vi "mul_add_24_dc_ht_rnd.vi"(8 "add":fxp<+/-,24,16> format="%#_10g", 10 "Signal":fxp<+/-,24,16>=32.0, 11 "coeff":fxp<+/-,18,2>=0.5) -> (1 "out":fxp<+/-,24,16>)   [LabVIEW 2018]
uses:
  <vilib>/rvi/FXPMathLib/basic elements/DSP48E/simVIs/niFpgaDsp48eSimulationState.ctl
  <vilib>/rvi/FXPMathLib/basic elements/DSP48E/subVIs/niFpgaDsp48eType.ctl
  <vilib>/rvi/FXPMathLib/basic elements/DSP48E/subVIs/niFpgaDsp48eAlumodeOpmodeCarryinselState.ctl
  <vilib>/rvi/FXPMathLib/basic elements/DSP48E/subVIs/niFpgaDsp48eUseMultiplierState.ctl
  <vilib>/rvi/FXPMathLib/basic elements/DSP48E/subVIs/niFpgaDsp48eLogicUnitModeState.ctl
  <vilib>/rvi/FXPMathLib/basic elements/DSP48E/subVIs/niFpgaDsp48eSelectPatternState.ctl
  <vilib>/rvi/FXPMathLib/basic elements/DSP48E/subVIs/niFpgaDsp48eSelectMaskState.ctl
  <vilib>/rvi/FXPMathLib/basic elements/DSP48E/subVIs/niFpgaDsp48eAutoresetState.ctl
  <vilib>/rvi/FXPMathLib/basic elements/DSP48E/simVIs/niFpgaDsp48eResets.ctl
  <vilib>/rvi/FXPMathLib/basic elements/DSP48E/simVIs/niFpgaDsp48eRegisters.ctl
  <vilib>/rvi/FXPMathLib/basic elements/DSP48E/simVIs/niFpgaDsp48eCheckMode.vi
  <vilib>/rvi/FXPMathLib/basic elements/DSP48E/simVIs/niFpgaDsp48eReportInvalidMode.vi
  <vilib>/rvi/FXPMathLib/basic elements/DSP48E/simVIs/niFpgaDsp48eSimBundleEnables.vi
  <vilib>/rvi/FXPMathLib/basic elements/DSP48E/simVIs/niFpgaDsp48eSimMultiplier.vi
  <vilib>/rvi/FXPMathLib/basic elements/DSP48E/simVIs/niFpgaDsp48eSimArithmetic.vi
  <vilib>/rvi/FXPMathLib/basic elements/DSP48E/simVIs/niFpgaDsp48eSimPatternDetect.vi
  <vilib>/rvi/FXPMathLib/basic elements/DSP48E/simVIs/niFpgaDsp48eSimP.vi
  <vilib>/rvi/FXPMathLib/basic elements/DSP48E/simVIs/niFpgaDsp48eSimUpdateState.vi
  <vilib>/rvi/FXPMathLib/basic elements/DSP48E/XNode/niFpgaDsp48e.xnode
panel:
  out "appended array 2":bool[](array[boolean])
  out "appended array":bool[](array[boolean])
  out "number":fxp<+/-,30,16>
  in  "Signal 2":fxp<+/-,24,16>=32.0
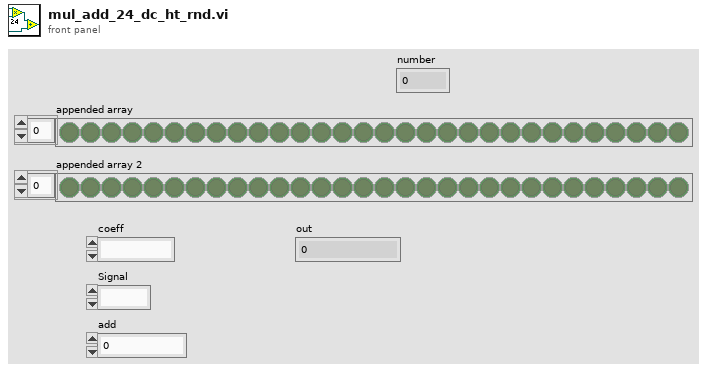
[diagram p1: front panel]
types:
  T1 = cluster{"Boolean array[0]":bool, "Boolean array[1]":bool, "Boolean array[2]":bool, "Boolean array[3]":bool, "Boolean array[4]":bool, "Boolean array[5]":bool, "Boolean array[6]":bool, "Boolean array[7]":bool, "Boolean array[8]":bool, "Boolean array[9]":bool, "Boolean array[10]":bool, "Boolean array[11]":bool, "Boolean array[12]":bool, "Boolean array[13]":bool, "Boolean array[14]":bool, "Boolean array[15]":bool, "Boolean array[16]":bool, "Boolean array[17]":bool, "Boolean array[18]":bool, "Boolean array[19]":bool, "Boolean array[20]":bool, "Boolean array[21]":bool, "Boolean array[22]":bool, "Boolean array[23]":bool}
  T2 = cluster{"Boolean array[0]":bool, "Boolean array[1]":bool, "Boolean array[2]":bool, "Boolean array[3]":bool, "Boolean array[4]":bool, "Boolean array[5]":bool, "Boolean array[6]":bool, "Boolean array[7]":bool, "Boolean array[8]":bool, "Boolean array[9]":bool, "Boolean array[10]":bool, "Boolean array[11]":bool, "Boolean array[12]":bool, "Boolean array[13]":bool, "Boolean array[14]":bool, "Boolean array[15]":bool, "Boolean array[16]":bool, "Boolean array[17]":bool}
  T3 = cluster{"Boolean array[0]":bool, "Boolean array[1]":bool, "Boolean array[2]":bool, "Boolean array[3]":bool, "Boolean array[4]":bool, "Boolean array[5]":bool, "Boolean array[6]":bool, "Boolean array[7]":bool, "Boolean array[8]":bool, "Boolean array[9]":bool, "Boolean array[10]":bool, "Boolean array[11]":bool, "Boolean array[12]":bool, "Boolean array[13]":bool, "Boolean array[14]":bool, "Boolean array[15]":bool, "Boolean array[16]":bool, "Boolean array[17]":bool, "Boolean array[18]":bool, "Boolean array[19]":bool, "Boolean array[20]":bool, "Boolean array[21]":bool, "Boolean array[22]":bool, "Boolean array[23]":bool, "Boolean array[24]":bool, "Boolean array[25]":bool, "Boolean array[26]":bool, "Boolean array[27]":bool, "Boolean array[28]":bool, "Boolean array[29]":bool, "Boolean array[30]":bool, "Boolean array[31]":bool, "Boolean array[32]":bool, "Boolean array[33]":bool, "Boolean array[34]":bool, "Boolean array[35]":bool, "Boolean array[36]":bool, "Boolean array[37]":bool, "Boolean array[38]":bool, "Boolean array[39]":bool, "Boolean array[40]":bool, "Boolean array[41]":bool, "Boolean array[42]":bool, "Boolean array[43]":bool, "Boolean array[44]":bool, "Boolean array[45]":bool, "Boolean array[46]":bool, "Boolean array[47]":bool}
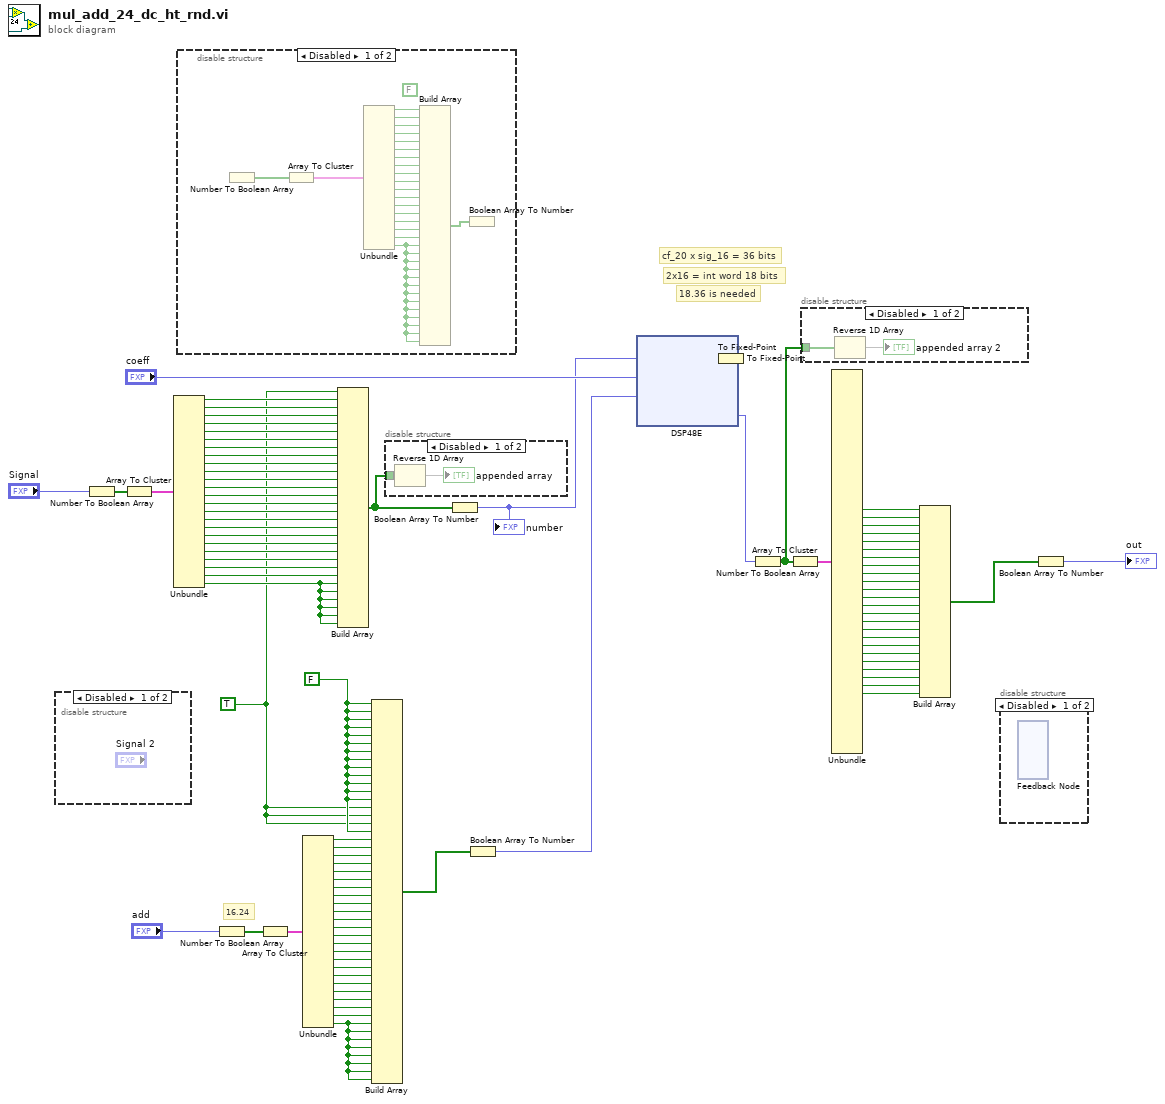
[diagram p0: block diagram]
diagram:
  w3 = TRUE ("Boolean array[0]")
  w4 = FALSE ("Boolean array[0]")
  # "16.24"
  # "18.36 is needed"
  # "2x16 = int word 18 bits"
  # "cf_20 x sig_16 = 36 bits"
  n1 = disable-structure shown="Disabled" {
    frame Disabled {
    }
    frame Enabled {
    }
  }
  n2 = Number To Boolean Array(number="Signal") -> (Boolean array=w28:bool[])
  n3 = Array To Cluster(array=w28) -> (cluster=w92:T1)
  n4 = Unbundle(w92) -> ("Boolean array[0]"=w26:bool, "Boolean array[1]"=w25:bool, "Boolean array[2]"=w24:bool, "Boolean array[3]"=w23:bool, "Boolean array[4]"=w22:bool, "Boolean array[5]"=w21:bool, "Boolean array[6]"=w91:bool, "Boolean array[7]"=w90:bool, "Boolean array[8]"=w89:bool, "Boolean array[9]"=w88:bool, "Boolean array[10]"=w87:bool, "Boolean array[11]"=w86:bool, "Boolean array[12]"=w85:bool, "Boolean array[13]"=w84:bool, "Boolean array[14]"=w83:bool, "Boolean array[15]"=w82:bool, "Boolean array[16]"=w45:bool, "Boolean array[17]"=w44:bool, "Boolean array[18]"=w39:bool, "Boolean array[19]"=w40:bool, "Boolean array[20]"=w41:bool, "Boolean array[21]"=w42:bool, "Boolean array[22]"=w43:bool, "Boolean array[23]"=w14:bool)
  n5 = disable-structure shown="Disabled" {
    frame Disabled {
      (unwired) FALSE ("Boolean array[0]")
      n6 = Number To Boolean Array() -> (Boolean array=w94:bool[])  [unwired: 1 in]
      n7 = Array To Cluster(array=w94) -> (cluster=w96:T2)
      n8 = Unbundle(w96) -> ("Boolean array[0]"=w97:bool, "Boolean array[1]"=w113:bool, "Boolean array[2]"=w98:bool, "Boolean array[3]"=w99:bool, "Boolean array[4]"=w100:bool, "Boolean array[5]"=w101:bool, "Boolean array[6]"=w102:bool, "Boolean array[7]"=w103:bool, "Boolean array[8]"=w104:bool, "Boolean array[9]"=w105:bool, "Boolean array[10]"=w106:bool, "Boolean array[11]"=w107:bool, "Boolean array[12]"=w108:bool, "Boolean array[13]"=w109:bool, "Boolean array[14]"=w110:bool, "Boolean array[15]"=w111:bool, "Boolean array[16]"=w112:bool, "Boolean array[17]"=w93:bool)
      n9 = Build Array(w97, w113, w98, w99, w100, w101, w102, w103, w104, w105, w106, w107, w108, w109, w110, w111, w112, w93, w93, w93, w93, w93, w93, w93, w93, w93, w93, w93, w93, w93) -> (w95:bool[])
      n10 = Boolean Array To Number(Boolean array=w95) -> ()  [unwired: 1 out]
    }
    frame Enabled {
    }
  }
  n11 = Number To Boolean Array(number="add") -> (Boolean array=w81:bool[])
  n12 = Array To Cluster(array=w81) -> (cluster=w80:T1)
  n13 = Unbundle(w80) -> ("Boolean array[0]"=w57:bool, "Boolean array[1]"=w58:bool, "Boolean array[2]"=w59:bool, "Boolean array[3]"=w60:bool, "Boolean array[4]"=w61:bool, "Boolean array[5]"=w62:bool, "Boolean array[6]"=w63:bool, "Boolean array[7]"=w64:bool, "Boolean array[8]"=w65:bool, "Boolean array[9]"=w66:bool, "Boolean array[10]"=w67:bool, "Boolean array[11]"=w68:bool, "Boolean array[12]"=w69:bool, "Boolean array[13]"=w70:bool, "Boolean array[14]"=w71:bool, "Boolean array[15]"=w72:bool, "Boolean array[16]"=w73:bool, "Boolean array[17]"=w74:bool, "Boolean array[18]"=w75:bool, "Boolean array[19]"=w76:bool, "Boolean array[20]"=w77:bool, "Boolean array[21]"=w78:bool, "Boolean array[22]"=w79:bool, "Boolean array[23]"=w5:bool)
  n14 = Build Array(w3, w26, w25, w24, w23, w22, w21, w91, w90, w89, w88, w87, w86, w85, w84, w83, w82, w45, w44, w39, w40, w41, w42, w43, w14, w14, w14, w14, w14, w14) -> (w16:bool[])
  n15 = Build Array(w4, w4, w4, w4, w4, w4, w4, w4, w4, w4, w4, w4, w4, w3, w3, w3, w4, w57, w58, w59, w60, w61, w62, w63, w64, w65, w66, w67, w68, w69, w70, w71, w72, w73, w74, w75, w76, w77, w78, w79, w5, w5, w5, w5, w5, w5, w5, w5) -> (w31:bool[])
  n16 = disable-structure shown="Disabled" {
    disable-tunnel: w16 -> [w115 _]
    frame Disabled {
      n17 = Reverse 1D Array(array=w115) -> (reversed array=→"appended array":bool[])
    }
    frame Enabled {
    }
  }
  n18 = Boolean Array To Number(Boolean array=w16) -> (number=w20:fxp<+/-,30,16>)
  "number" <- w20
  n19 = Boolean Array To Number(Boolean array=w31) -> (number=w6:fxp<+/-,48,18>)
  n20 = To Fixed-Point(number=w20) -> (fixed-point=w1:fxp<+/-,30,16>)  [unwired: 1 in]
  n21 = To Fixed-Point(number=w1) -> (fixed-point=w2:fxp<+/-,25,11>)  [unwired: 1 in]
  n22 = xnode ("DSP48E")("a"=w2, "b"="coeff", "c"=w6) -> ("p"=w38:fxp<+/-,48,48>)
  n23 = Number To Boolean Array(number=w38) -> (Boolean array=w15:bool[])
  n24 = Array To Cluster(array=w15) -> (cluster=w56:T3)
  n25 = disable-structure shown="Disabled" {
    disable-tunnel: w15 -> [w116 _]
    frame Disabled {
      n26 = Reverse 1D Array(array=w116) -> (reversed array=→"appended array 2":bool[])
    }
    frame Enabled {
    }
  }
  n27 = Unbundle(w56) -> ("Boolean array[17]"=w13:bool, "Boolean array[18]"=w12:bool, "Boolean array[19]"=w11:bool, "Boolean array[20]"=w10:bool, "Boolean array[21]"=w9:bool, "Boolean array[22]"=w8:bool, "Boolean array[23]"=w7:bool, "Boolean array[24]"=w49:bool, "Boolean array[25]"=w50:bool, "Boolean array[26]"=w51:bool, "Boolean array[27]"=w52:bool, "Boolean array[28]"=w53:bool, "Boolean array[29]"=w54:bool, "Boolean array[30]"=w55:bool, "Boolean array[31]"=w46:bool, "Boolean array[32]"=w47:bool, "Boolean array[33]"=w48:bool, "Boolean array[34]"=w37:bool, "Boolean array[35]"=w36:bool, "Boolean array[36]"=w30:bool, "Boolean array[37]"=w29:bool, "Boolean array[38]"=w18:bool, "Boolean array[39]"=w19:bool, "Boolean array[40]"=w17:bool)  [unwired: 24 out]
  n28 = Build Array(w13, w12, w11, w10, w9, w8, w7, w49, w50, w51, w52, w53, w54, w55, w46, w47, w48, w37, w36, w30, w29, w18, w19, w17) -> (w35:bool[])
  n29 = disable-structure shown="Disabled" {
    frame Disabled {
      n30 = feedback #1() -> ()  [unwired: 2 in]
      n31 = feedback-in #1() -> ()  [unwired: 1 in, 1 out]
    }
    frame Enabled {
    }
  }
  n32 = Boolean Array To Number(Boolean array=w35) -> (number=→"out":fxp<+/-,24,16>)
